vi "TimeShiftDataSubMean.vi"(5 "ZoneLength":sgl[](array[numeric]), 6 "bits A/D":u16=8, 7 "Filter":T1, 8 "output cluster":T2, 9 "Array In":i16[][](array[numeric])) -> (3 "Sat Pts":i32, 4 "Array Out":i16[][](array[numeric]))   [LabVIEW 2022 SP3]
uses:
  <vilib>/Analysis/NI_AALPro.lvlib
  <vilib>/gmath/NI_Gmath.lvlib
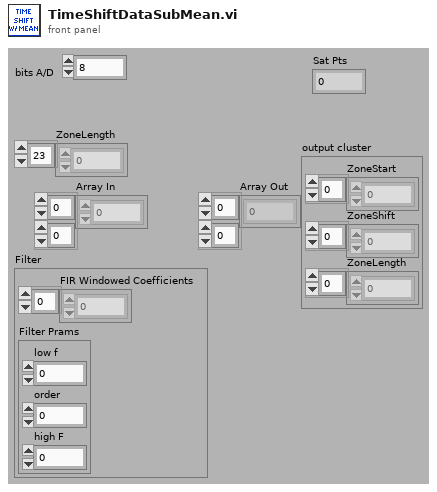
[diagram p1: front panel]
types:
  T1 = cluster{"FIR Windowed Coefficients":dbl[], "Filter Prams":cluster{"low f":i32, "order":i32, "high F":i32}}
  T2 = cluster{"ZoneStart":sgl[], "ZoneShift":dbl[], "ZoneLength":sgl[]}
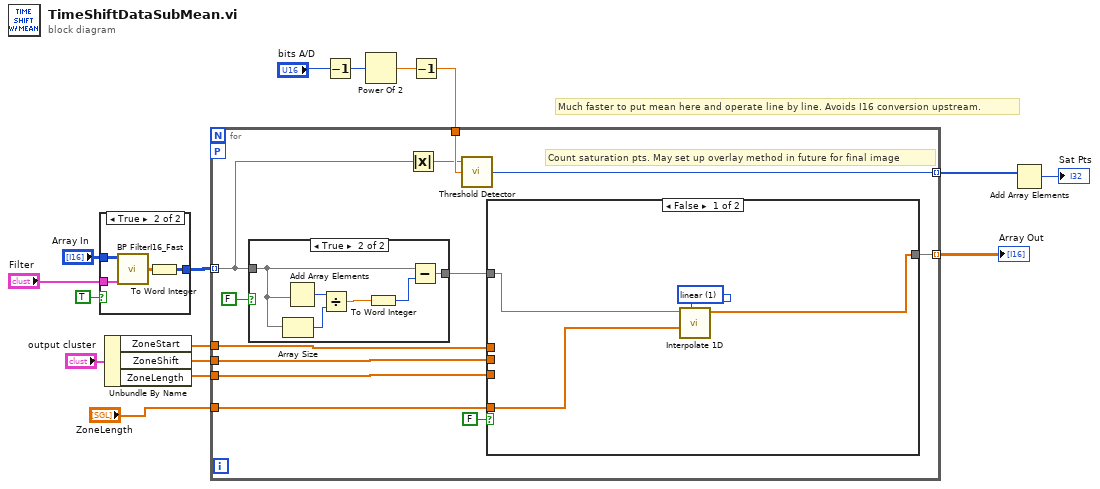
[diagram p0: block diagram]
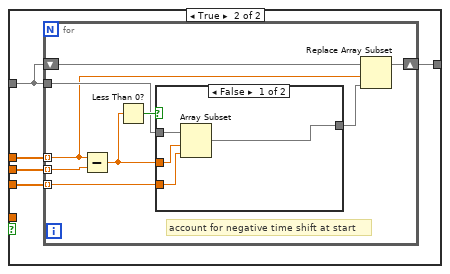
[diagram p3: hidden frame]
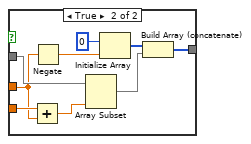
[diagram p4: hidden frame]
diagram:
  # "Much faster to put mean here and operate line by line. Avoids I16 conversion upstream."
  n1 = case shown="True" TRUE {
    tunnel: "Array In" -> [w17 w21]
    tunnel: [w17 w18] -> w8
    tunnel: "Filter" -> [_ w19]
    frame False {
    }
    frame True {
      n2 = call "BP FilterI16_Fast.vi"("Filter"=w19, "Array in"=w21) -> ("Filtered X"=w20:dbl[][])  [unwired: 4 in]
      n3 = To Word Integer(number=w20) -> (16bit integer=w18:i16[][])
    }
  }
  n4 = Unbundle By Name("output cluster") -> ("ZoneStart"=w14:sgl[], "ZoneShift"=w13:dbl[], "ZoneLength"=w12:sgl[])
  n5 = Decrement(x="bits A/D") -> (x-1=w4:u16)
  n6 = Power Of 2(x=w4) -> (2^x=w3:dbl)
  n7 = Decrement(x=w3) -> (x-1=w2:dbl)
  n8 = for {
    tunnel: w8 -> [w24] mode=indexing
    tunnel: w14 -> [w33]
    tunnel: w13 -> [w32]
    tunnel: w12 -> [w31]
    tunnel: [w30] -> w16 mode=indexing
    tunnel: w2 -> [w29]
    tunnel: [w26] -> w11 mode=indexing
    tunnel: "ZoneLength" -> [w22]
    workers-P: _ -> [_]
    # "Count saturation pts. May set up overlay method in future for final image"
    n9 = case shown="True" FALSE {
      tunnel: [w65 w71] -> w27
      tunnel: w24 -> [w65 w70]
      frame False {
      }
      frame True {
        n10 = Array Size(array=w70) -> (size(s)=w67:i32)
        n11 = Add Array Elements(numeric array=w70) -> (sum=w69:i16)
        n12 = Divide(x=w69, y=w67) -> (x/y=w68:dbl)
        n13 = To Word Integer(number=w68) -> (16bit integer=w66:i16)
        n14 = Subtract(x=w70, y=w66) -> (x-y=w71:i16[])
      }
    }
    n15 = Absolute Value(x=w24) -> (abs(x)=w28:i16[])
    n16 = call <vilib>:"Threshold Detector.vi"("threshold"=w29, "X"=w28) -> ("count"=w26:i32)  [unwired: 1 in, 2 out]
    n17 = case shown="False" FALSE {
      tunnel: w33 -> [_ w42]
      tunnel: w32 -> [_ w41]
      tunnel: w31 -> [_ w40]
      tunnel: [w35 w39] -> w30
      tunnel: w27 -> [w36 w38]
      tunnel: w22 -> [w34 _]
      frame False {
        w37 = 1 items=["nearest", "linear", "spline", "cubic Hermite", "Lagrange"] ("method")
        n18 = call <vilib>:"Interpolate 1D.vi"("method"=w37, "xi"=w34, "Y"=w36) -> ("yi"=w35:dbl[])  [unwired: 6 in, 2 out]
      }
      frame True {
        n19 = for {
          tunnel: w42 -> [w44] mode=indexing
          tunnel: w40 -> [w51] mode=indexing
          tunnel: w41 -> [w50] mode=indexing
          tunnel: w38 -> [w47]
          shift-right: [w46] -> w39
          shift-left: w38 -> [w45]
          # "account for negative time shift at start"
          n20 = Subtract(x=w44, y=w50) -> (x-y=w48:dbl)
          n21 = Less Than 0?(x=w48) -> (x < 0?=w49:bool)
          n22 = case shown="False" w49 {
            tunnel: w47 -> [w55 w63]
            tunnel: w51 -> [w53 w64]
            tunnel: [w54 w58] -> w43
            tunnel: w48 -> [w52 w61]
            frame False {
              n23 = Array Subset(array=w55, index=w52, length=w53) -> (w54:i16[])
            }
            frame True {
              n24 = Add(x=w64, y=w61) -> (x+y=w57:dbl)
              n25 = Negate(x=w61) -> (-x=w56:dbl)
              n26 = Array Subset(array=w63, length=w57) -> (w59:i16[])  [unwired: 1 in]
              n27 = Initialize Array(i16 0, w56) -> (w60:i16[])
              n28 = Build Array (concatenate)(w60, w59) -> (w58:i16[])
            }
          }
          n29 = Replace Array Subset(array=w45, new element=w43, index=w44) -> (w46:i16[])
        }
      }
    }
  }
  "Array Out" <- w16
  n30 = Add Array Elements(numeric array=w11) -> (sum=→"Sat Pts":i32)
